vi "AMQP_credentials.vi"() -> ()   [LabVIEW 2016]
panel:
  in  "password":string
  in  "username":string
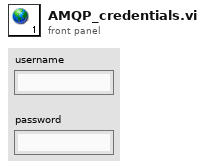
[diagram p1: front panel]
diagram:
